vi "2event_struct_ineinander.vi"() -> ()   [LabVIEW 2013]
panel:
  out "Numerisch":dbl
  in  "addiere 1":bool
  out "langsames Ding is zumindest einmal geloffen?":bool
  out "Notaus Ja?":bool
  in  "Stopp aeussere Schleife":bool
  out "ohmeingottohmeingottohmeingott":bool
  out "langsames Ding laeuft":bool
  in  "langsames Ding stoppen":bool
  in  "Stopp innere Schleife":bool
  in  "Notaus":bool
  in  "langsam":bool
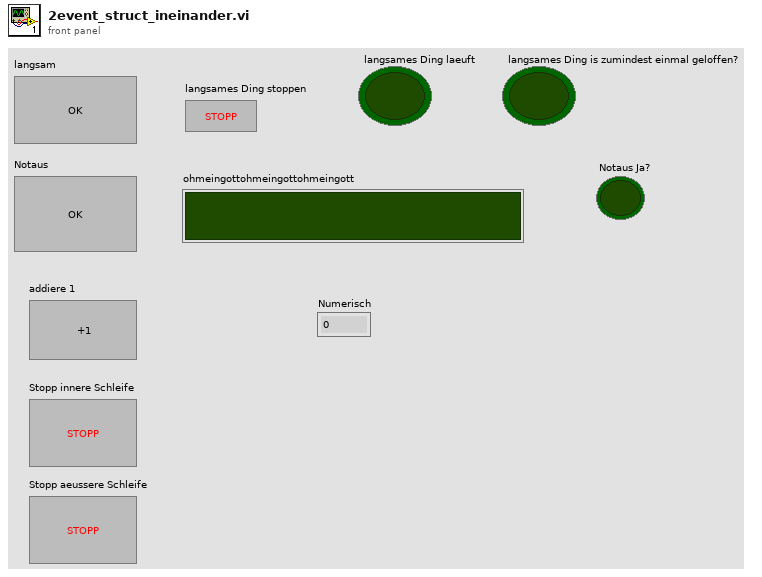
[diagram p1: front panel]
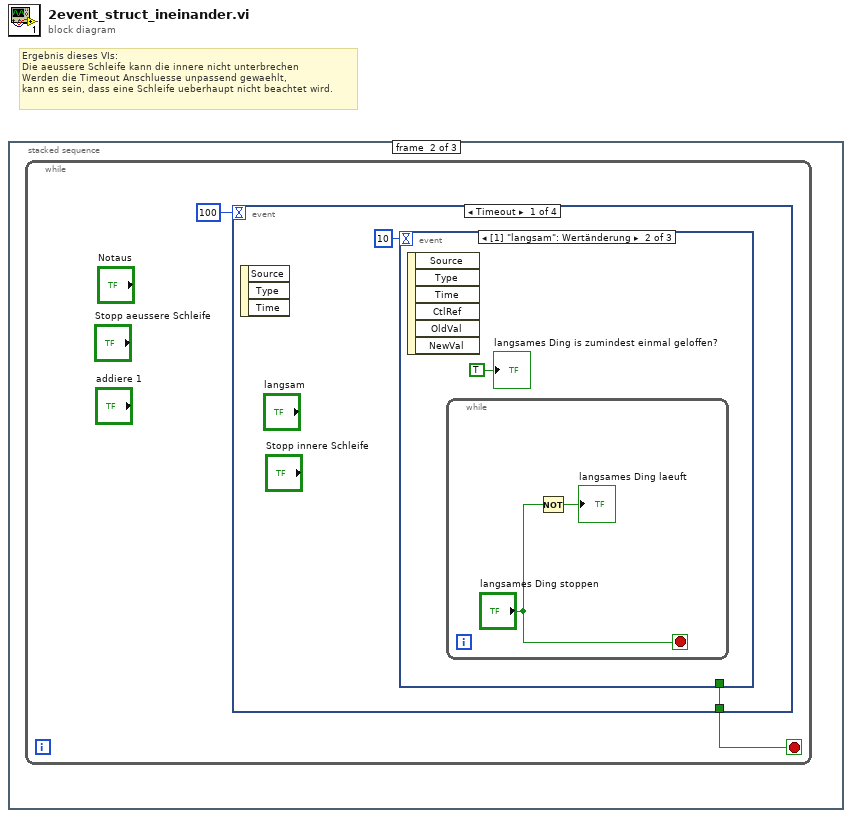
[diagram p0: block diagram]
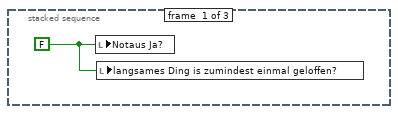
[diagram p2: hidden frame]
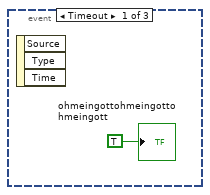
[diagram p3: hidden frame]
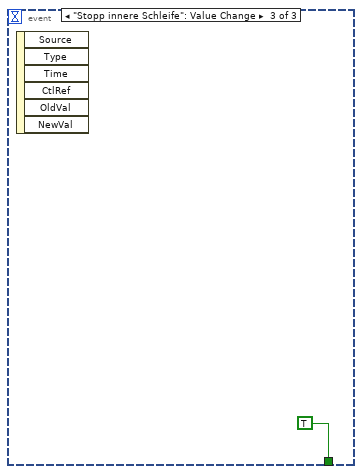
[diagram p4: hidden frame]
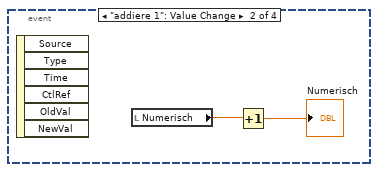
[diagram p5: hidden frame]
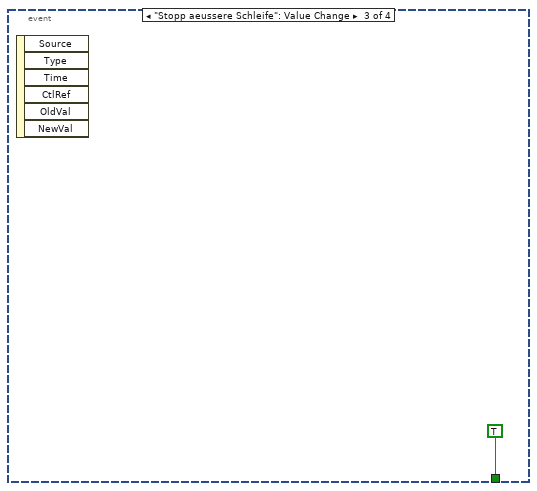
[diagram p6: hidden frame]
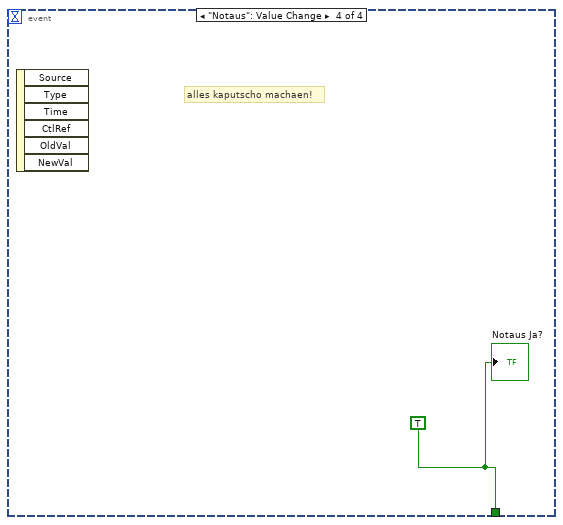
[diagram p7: hidden frame]
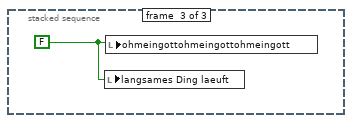
[diagram p8: hidden frame]
diagram:
  # "Ergebnis dieses VIs:\nDie aeussere Schleife kann die innere nicht unterbrechen\nWerden die Timeout Anschluesse unpassend gewaehlt, \nkann es sein, dass eine Schleife ueberhaupt nicht beachtet wird."
  n1 = stacked-sequence {
    frame #0 {
      w1 = FALSE
      n2 = local write "Notaus Ja?"(w1) -> ()
      n3 = local write "langsames Ding is zumindest einmal geloffen?"(w1) -> ()
    }
    frame #1 {
      n4 = while {
        stop <- w3 stop-if-true
        n5 = event shown="[0] Timeout" {
          selector: _ -> [_ _ _ _]
          dyn-events: _ -> [_ _ _ _]
          timeout: 100 -> [_ _ _ _]
          tunnel: [w4 _ TRUE w14] -> w3
          event Timeout {
            n6 = event-data() -> ()  [unwired: 1 in, 3 out]
            n7 = event shown="[1] \"langsam\": Wertänderung" {
              selector: _ -> [_ _ _]
              dyn-events: _ -> [_ _ _]
              timeout: 10 -> [_ _ _]
              tunnel: [_ _ TRUE] -> w4
              event Timeout {
                n8 = event-data() -> ()  [unwired: 1 in, 3 out]
                "ohmeingottohmeingottohmeingott" <- TRUE
              }
              event "langsam": Value Change {
                n9 = event-data() -> ()  [unwired: 1 in, 6 out]
                n10 = while {
                  stop <- "langsames Ding stoppen" stop-if-true
                  n11 = Not(x="langsames Ding stoppen") -> (.not. x?=→"langsames Ding laeuft":bool)
                }
                "langsames Ding is zumindest einmal geloffen?" <- TRUE ("langsames Ding is zumindest einmal geloffen")
              }
              event "Stopp innere Schleife": Value Change {
                n12 = event-data() -> ()  [unwired: 1 in, 6 out]
              }
            }
          }
          event "addiere 1": Value Change {
            n13 = event-data() -> ()  [unwired: 1 in, 6 out]
            n14 = local read "Numerisch"() -> (w11:dbl)
            n15 = Increment(x=w11) -> (x+1=→"Numerisch":dbl)
          }
          event "Stopp aeussere Schleife": Value Change {
            n16 = event-data() -> ()  [unwired: 1 in, 6 out]
          }
          event "Notaus": Value Change {
            w14 = TRUE
            # "alles kaputscho machaen!"
            n17 = event-data() -> ()  [unwired: 1 in, 6 out]
            "Notaus Ja?" <- w14
          }
        }
      }
    }
    frame #2 {
      w15 = FALSE
      n18 = local write "langsames Ding laeuft"(w15) -> ()
      n19 = local write "ohmeingottohmeingottohmeingott"(w15) -> ()
    }
  }
